vi "GFITS_imnameExtension.vi"(9 "imname in":string) -> (1 "rootname (no extension)":string, 2 "imname out":string)   [LabVIEW 2016]
panel:
  in  "extension to look":string="fits"
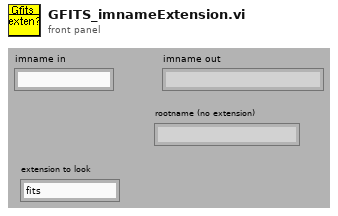
[diagram p1: front panel]
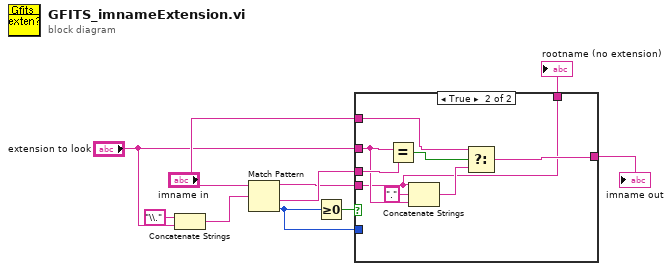
[diagram p0: block diagram]
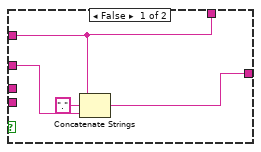
[diagram p2: hidden frame]
diagram:
  n1 = Concatenate Strings("\\." ("string"), "extension to look") -> (w1:string)
  n2 = Match Pattern(string="imname in", regular expression=w1) -> (before substring=w5:string, after substring=w8:string, offset past match=w9:i32)  [unwired: 2 out]
  n3 = Greater Or Equal To 0?(x=w9) -> (x >= 0?=w10:bool)
  n4 = case shown="True" w10 {
    tunnel: w9 -> [_ _]
    tunnel: w8 -> [_ w22]
    tunnel: "extension to look" -> [w13 w17]
    tunnel: "imname in" -> [w11 w20]
    tunnel: [w12 w19] -> w6
    tunnel: w5 -> [_ w15]
    tunnel: [w11 w15] -> w4
    frame False {
      n5 = Concatenate Strings(w11, "." ("string"), w13) -> (w12:string)
    }
    frame True {
      n6 = Equal?(x=w17, y=w22) -> (x = y?=w21:bool)
      n7 = Concatenate Strings(w15, "." ("string"), w17) -> (w16:string)
      n8 = Select(t=w20, s=w21, f=w16) -> (s? t:f=w19:string)
    }
  }
  "imname out" <- w6
  "rootname (no extension)" <- w4
